vi "ma_Calculate window.vi"(6 "scaled for":enum16{"DC", "RMS"}(ring), 10 "array size":i32, 11 "window":T1(ring)=enum."Hanning") -> (3 "Window data":dbl[](array[numeric]) format="%0.2f")   [LabVIEW 2020, in "NI_MAPro.lvlib"]
uses:
  NI_MAPro.lvlib
  AllCosWindow (DBL).vi
  NI_AALPro.lvlib
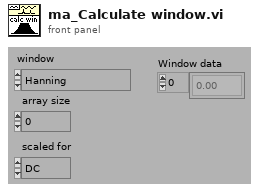
[diagram p1: front panel]
types:
  T1 = enum16{"Rectangular (none)", "Hanning", "Low side lobe"}
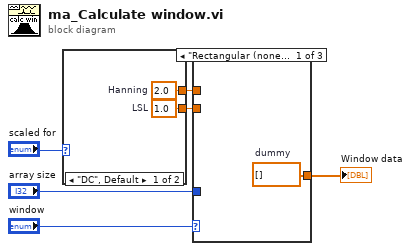
[diagram p0: block diagram]
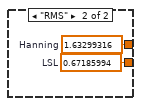
[diagram p2: hidden frame]
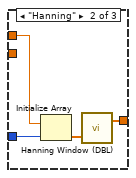
[diagram p3: hidden frame]
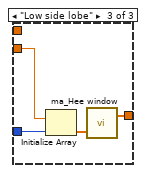
[diagram p4: hidden frame]
diagram:
  n1 = case shown="\"DC\", Default" "scaled for" {
    tunnel: [w8 w10] -> w3
    tunnel: [w7 w9] -> w2
    frame "DC", Default {
      w7 = 1.0  # LSL
      w8 = 2.0  # Hanning
    }
    frame "RMS" {
      w9 = 0.67185994  # LSL
      w10 = 1.63299316  # Hanning
    }
  }
  n2 = case shown="\"Rectangular (none)\", Default" "window" {
    tunnel: "array size" -> [_ w15 w19]
    tunnel: w3 -> [_ w14 _]
    tunnel: [w11 w12 w17] -> w1
    tunnel: w2 -> [_ _ w16]
    frame "Rectangular (none)", Default {
      w11 = dbl[] []  # dummy
    }
    frame "Hanning" {
      n3 = Initialize Array(w14, w15) -> (w13:dbl[])
      n4 = call "Hanning Window (DBL).vi"("X"=w13) -> ("Windowed X"=w12:dbl[])  [unwired: 1 out]
    }
    frame "Low side lobe" {
      n5 = Initialize Array(w16, w19) -> (w18:dbl[])
      n6 = call "ma_Hee window.vi"("X"=w18) -> ("Hee {X}"=w17:dbl[])  [unwired: 1 out]
    }
  }
  "Window data" <- w1
